vi "Ref Read.vi"(4 "error in (no error)":errorcluster, 6 "Container State":T4, 7 "Display State In":T1={"Prompt"="Click to add", "Listbox"=refnum, "Required"={"Strings"=[], "Bottom"=FALSE, "Italic"=FALSE, "FG"=0, "BG"=16777215, "Bold"=FALSE}, "Items"=[], "Req'd"=[], "Events"={"Items Changed"=refnum, "List Changed"=refnum}, "Max Rows"=-1, "Default name"=""}) -> (0 "error out":errorcluster, 2 "Value":refnum<vi>, 3 "Display State Out":T1={"Prompt"="Click to add", "Listbox"=refnum, "Required"={"Strings"=[], "Bottom"=FALSE, "Italic"=FALSE, "FG"=0, "BG"=16777215, "Bold"=FALSE}, "Items"=[], "Req'd"=[], "Events"={"Items Changed"=refnum, "List Changed"=refnum}, "Max Rows"=-1, "Default name"=""})   [LabVIEW 2015, in "KListboxEx.xctl"]
uses:
  KListboxEx.xctl
  <vilib>/_xctls/Container State.ctl
  State.ctl
  Required.ctl
  Events.ctl
  Event Action.ctl
  <vilib>/_xctls/XControlSupport.lvlib
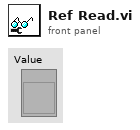
[diagram p1: front panel]
types:
  T1 = typedef "KListboxEx.xctl/State.ctl" = cluster{"Prompt":string, "Listbox":refnum<vi>, "Required":T2, "Items":string[], "Req'd":bool[], "Events":T3, "Max Rows":i32, "Default name":string}
  T2 = typedef "KListboxEx.xctl/Required.ctl" = cluster{"Strings":string[], "Bottom":bool, "Italic":bool, "FG":u32, "BG":u32, "Bold":bool}
  T3 = typedef "KListboxEx.xctl/Events.ctl" = cluster{"Items Changed":refnum<user-event>, "List Changed":refnum<user-event>}
  T4 = typedef "XControlSupport.lvlib/Container State.ctl" = cluster{"Indicator?":bool, "Run Mode?":bool, " Refnum":refnum<vi>}
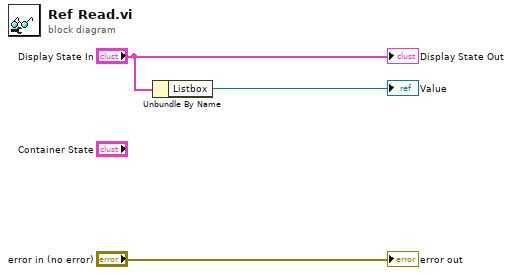
[diagram p0: block diagram]
diagram:
  n1 = Unbundle By Name("Display State In") -> ("Listbox"=→"Value":refnum<vi>)
  "error out" <- "error in (no error)"
  "Display State Out" <- "Display State In"
